vi "Read Flow Averaging Cycle Results.vi"(8 "error in (no error)":errorcluster, 11 "VISA resource name":refnum<visa-resource-name>) -> (0 "error out":errorcluster, 1 "MFC Voltage or Current":dbl, 2 "Flow Stability":bool, 3 "VISA resource name out":refnum<visa-resource-name>, 4 "MFC Voltage or Current Average":dbl, 5 "Flow Measurements":T1)   [LabVIEW 2023, in "Fluke Molbox 1 Plus.lvlib"]
doc: "Reads the results of a completed flow averaging cycle. If the cycle is aborted before it is completed, then the data will be lost."
uses:
  Fluke Molbox 1 Plus.lvlib
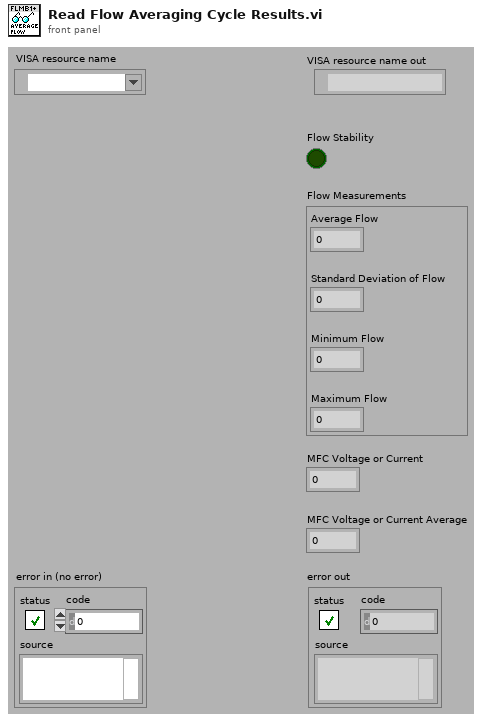
[diagram p1: front panel]
types:
  T1 = cluster{"Maximum Flow":dbl, "Minimum Flow":dbl, "Standard Deviation of Flow":dbl, "Average Flow":dbl}
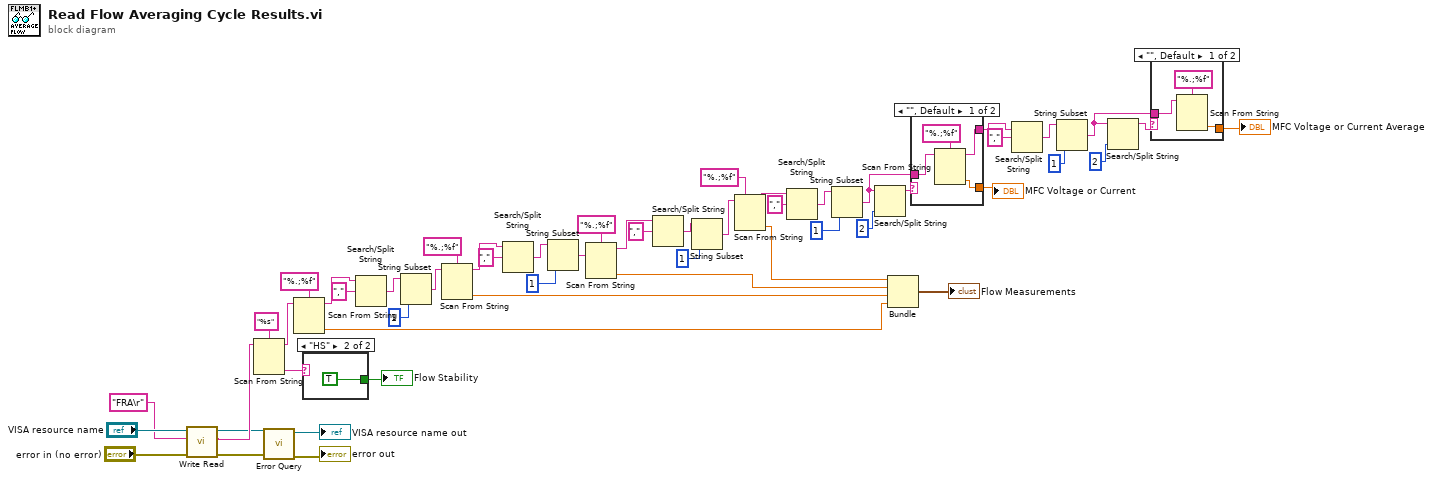
[diagram p0: block diagram]
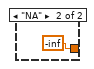
[diagram p2: hidden frame]
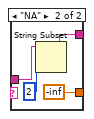
[diagram p3: hidden frame]
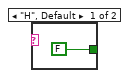
[diagram p4: hidden frame]
diagram:
  n1 = call "Write Read.vi"("error in (no error)"="error in (no error)", "Write String"="FRA\r" ("write buffer"), "VISA resource name"="VISA resource name") -> ("error out"=w2:errorcluster, "Read Response"=w5:string, "VISA resource name out"=w1:refnum<visa-resource-name>)  [unwired: 6 in]
  n2 = Scan From String(format string="%s", input string=w5) -> (remaining string=w46:string, output 1=w51:string)  [unwired: 3 in, 2 out]
  n3 = call "Error Query.vi"("error in (no error)"=w2, "VISA resource name"=w1) -> ("error out"=→"error out":errorcluster, "VISA resource name out"=→"VISA resource name out":refnum<visa-resource-name>)  [unwired: 6 in, 2 out]
  n4 = Scan From String(format string="%.;%f", input string=w46) -> (remaining string=w14:string, output 1=w19:dbl)  [unwired: 3 in, 2 out]
  n5 = case shown="\"HS\"" w51 {
    tunnel: [FALSE TRUE] -> w50
    frame "H", Default {
    }
    frame "HS" {
    }
  }
  "Flow Stability" <- w50
  n6 = Search/Split String(string=w14, search string/char (-)=",") -> (match + rest of string=w16:string)  [unwired: 1 in, 2 out]
  n7 = String Subset(string=w16, offset (0)=1) -> (substring=w12:string)  [unwired: 1 in]
  n8 = Scan From String(format string="%.;%f", input string=w12) -> (remaining string=w11:string, output 1=w10:dbl)  [unwired: 3 in, 2 out]
  n9 = Search/Split String(string=w11, search string/char (-)=",") -> (match + rest of string=w35:string)  [unwired: 1 in, 2 out]
  n10 = String Subset(string=w35, offset (0)=1) -> (substring=w33:string)  [unwired: 1 in]
  n11 = Scan From String(format string="%.;%f", input string=w33) -> (remaining string=w44:string, output 1=w20:dbl)  [unwired: 3 in, 2 out]
  n12 = Search/Split String(string=w44, search string/char (-)=",") -> (match + rest of string=w42:string)  [unwired: 1 in, 2 out]
  n13 = String Subset(string=w42, offset (0)=1) -> (substring=w40:string)  [unwired: 1 in]
  n14 = Scan From String(format string="%.;%f", input string=w40) -> (remaining string=w9:string, output 1=w21:dbl)  [unwired: 3 in, 2 out]
  n15 = Search/Split String(string=w9, search string/char (-)=",") -> (match + rest of string=w38:string)  [unwired: 1 in, 2 out]
  n16 = String Subset(string=w38, offset (0)=1) -> (substring=w30:string)  [unwired: 1 in]
  n17 = Search/Split String(string=w30, offset (0)=2) -> (substring before match=w31:string)  [unwired: 1 in, 2 out]
  n18 = Bundle(w21, w20, w10, w19) -> (→"Flow Measurements":cluster{dbl, dbl, dbl, dbl})  [unwired: 1 in]
  n19 = case shown="\"\", Default" w31 {
    tunnel: [w57 -inf ("Negative Infinity")] -> w47
    tunnel: w30 -> [w56 w60]
    tunnel: [w55 w61] -> w23
    frame "", Default {
      n20 = Scan From String(format string="%.;%f", input string=w56) -> (remaining string=w55:string, output 1=w57:dbl)  [unwired: 3 in, 2 out]
    }
    frame "NA" {
      n21 = String Subset(string=w60, offset (0)=2) -> (substring=w61:string)  [unwired: 1 in]
    }
  }
  "MFC Voltage or Current" <- w47
  n22 = Search/Split String(string=w23, search string/char (-)=",") -> (match + rest of string=w28:string)  [unwired: 1 in, 2 out]
  n23 = String Subset(string=w28, offset (0)=1) -> (substring=w24:string)  [unwired: 1 in]
  n24 = Search/Split String(string=w24, offset (0)=2) -> (substring before match=w25:string)  [unwired: 1 in, 2 out]
  n25 = case shown="\"\", Default" w25 {
    tunnel: [w64 -inf ("Negative Infinity")] -> w22
    tunnel: w24 -> [w63 _]
    frame "", Default {
      n26 = Scan From String(format string="%.;%f", input string=w63) -> (output 1=w64:dbl)  [unwired: 3 in, 3 out]
    }
    frame "NA" {
    }
  }
  "MFC Voltage or Current Average" <- w22
